vi "Trigger-simulation.vi"(8 "error in (no error)":errorcluster, 9 "Wakeup Reason":T1, 10 "Config. params. ref. in":refnum<data-value>, 11 "Acquis. params. ref. in":refnum<data-value>) -> (0 "error out":errorcluster, 1 "Tigger ok?":bool, 2 "Config. params. ref.":refnum<data-value>, 3 "Acquis. params. ref.":refnum<data-value>)   [LabVIEW 2013, in "CameraVision.lvlib" / "CV-Acquisition.lvclass"]
uses:
  CV-Acquisition.lvclass
  Configuration/CV-Configuration.lvclass
  <vilib>/Platform/TimedLoop/XDataNode/wakeup.ctl
  CV-Acquisition.lvclass/CV-Acquisition.ctl
  <vilib>/DAQmx/read.llb/DAQmx Read (Digital Bool 1Line 1Point).vi
  Read Gate when.vi
  Read Gate source.vi
  Read Trigger mode.vi
  <vilib>/DAQmx/miscellaneous.llb/DAQmx Fill In Error Info.vi
  <vilib>/Platform/TimedLoop/XDataNode/XDNodeRunTimeDep.lvlib
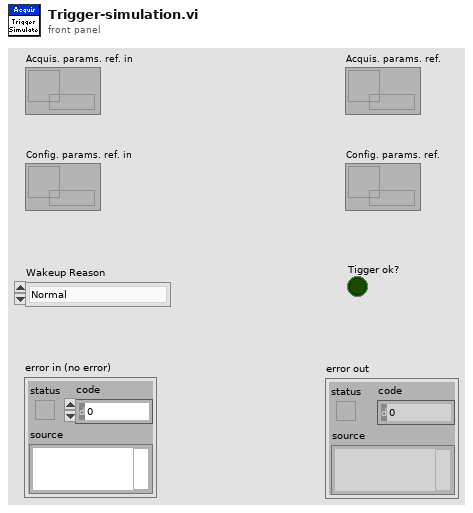
[diagram p1: front panel]
types:
  T1 = typedef "XDNodeRunTimeDep.lvlib/wakeup.ctl" = enum32{"Normal", "Aborted", "Asynchronous wakeup", "Timing source error", "Timed loop error", "Timeout"}
  T2 = typedef "CameraVision.lvlib/Acquisition.lvclass/Trigger-modes.ctl" = enum16{"Camera timed (not sync.)", "Framegrabber timed (sync.)", "Software timed (sync.)", "External timing (sync.)", "Manual (sync.)", "Gated - camera (not sync.)", "Gated - grabber (sync.)", "Gated - software (sync.)", "Gated - external (sync.)"}
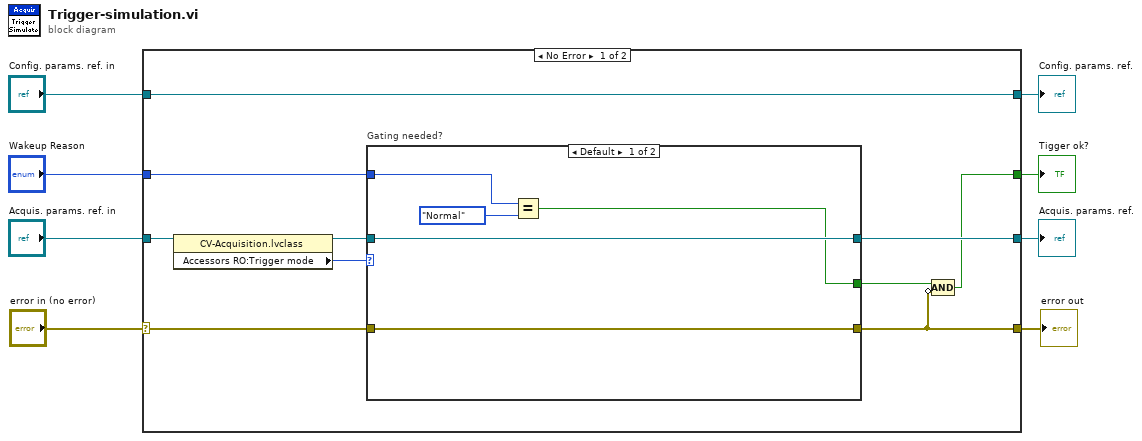
[diagram p0: block diagram]
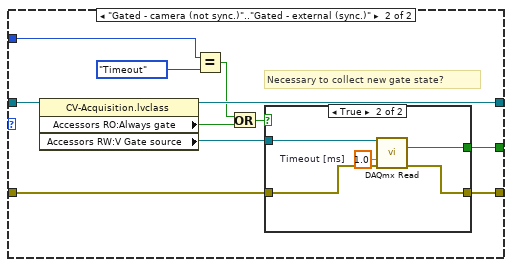
[diagram p2: hidden frame]
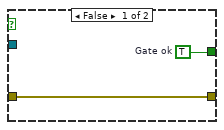
[diagram p3: hidden frame]
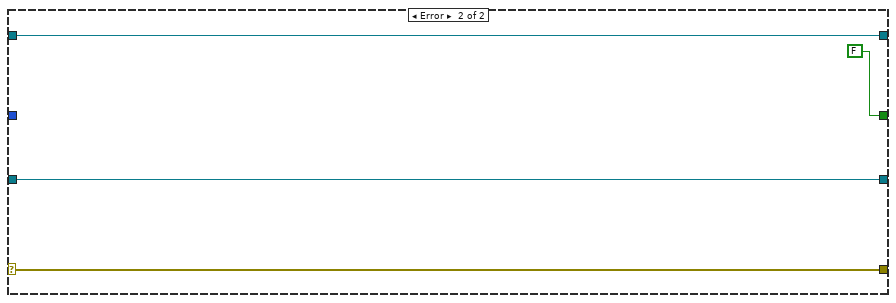
[diagram p4: hidden frame]
diagram:
  n1 = case shown="No Error" "error in (no error)" {
    selector: "error in (no error)" -> [w15 w45]
    tunnel: [w9 w45] -> w7
    tunnel: "Acquis. params. ref. in" -> [w18 w43]
    tunnel: [w13 w43] -> w3
    tunnel: [w10 w44] -> w4
    tunnel: "Config. params. ref. in" -> [w10 w44]
    tunnel: [w12 FALSE] -> w2
    tunnel: "Wakeup Reason" -> [w11 _]
    frame No Error {
      n2 = property class="CV-Acquisition.lvclass"(reference=w18) -> (reference out=w16:refnum<data-value>, "Accessors RO:Trigger mode"=w17:T2)  [unwired: 1 in, 1 out]
      n3 = case "Gating needed?" shown="Default" w17 {
        tunnel: w16 -> [w22 w34]
        tunnel: w15 -> [w23 w33]
        tunnel: [w23 w32] -> w9
        tunnel: [w19 w31] -> w14
        tunnel: [w22 w30] -> w13
        tunnel: w11 -> [w20 w28]
        frame Default {
          n4 = Equal?(x=w20, y=wakeup."Normal") -> (x = y?=w19:bool)
        }
        frame "Gated - camera (not sync.)".."Gated - external (sync.)" {
          # "Necessary to collect new gate state?"
          n5 = property class="CV-Acquisition.lvclass"(reference=w34) -> (reference out=w30:refnum<data-value>, "Accessors RO:Always gate"=w25:bool, "Accessors RW:V Gate source"=w29:refnum<k21>)  [unwired: 1 in, 1 out]
          n6 = Equal?(x=w28, y=wakeup."Timeout") -> (x = y?=w26:bool)
          n7 = Or(x=w26, y=w25) -> (x .or. y?=w24:bool)
          n8 = case shown="True" w24 {
            tunnel: w33 -> [w35 w40]
            tunnel: [w35 w39] -> w32
            tunnel: [w36 w38] -> w31
            tunnel: w29 -> [_ w37]
            frame False {
              w36 = TRUE  # Gate ok
            }
            frame True {
              w41 = 1.0  # Timeout [ms]
              n9 = call-poly <vilib>:"DAQmx Read.vi"("task/channels in"=w37, "timeout"=w41, "error in"=w40) -> ("data"=w38:bool, "error out"=w39:errorcluster)  [unwired: 10 in, 1 out]
            }
          }
        }
      }
      n10 = Compound Arithmetic op=AND(w14, invert w9) -> (w12:bool)
    }
    frame Error {
    }
  }
  "error out" <- w7
  "Acquis. params. ref." <- w3
  "Config. params. ref." <- w4
  "Tigger ok?" <- w2
